vi "Count VarINT.vi"(3 "Buffer":u8[](array[numeric])) -> (1 "Bytes":i32)   [LabVIEW 2020, in "Protobuf RAW.lvlib"]
uses:
  Protobuf RAW.lvlib
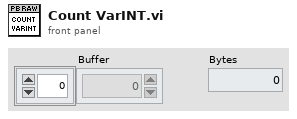
[diagram p1: front panel]
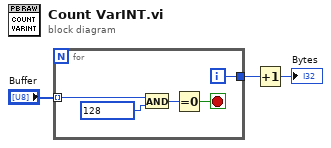
[diagram p0: block diagram]
diagram:
  n1 = for {
    tunnel: "Buffer" -> [w5] mode=indexing
    tunnel: [w4] -> w2
    i -> [w4]
    stop <- w6 stop-if-true
    n2 = And(x=w5, y=u8 128) -> (x .and. y?=w7:u8)
    n3 = Equal To 0?(x=w7) -> (x = 0?=w6:bool)
  }
  n4 = Increment(x=w2) -> (x+1=→"Bytes":i32)
